vi "Iman.vi"() -> ()   [LabVIEW 2017]
uses:
  <vilib>/myRIO/Instrument Drivers/Onboard IO/DIO/typedefs/DIO Reference.ctl
  <vilib>/myRIO/Common/Instrument Driver Framework/Utilities/typedefs/myRIO Generic Hardware Reference.ctl
  <vilib>/myRIO/Common/Instrument Driver Framework/Utilities/typedefs/Hardware Version Enum.ctl
  <vilib>/myRIO/Common/Instrument Driver Framework/Utilities/typedefs/myRIO v1.0 Reference.ctl
  <vilib>/myRIO/Common/Instrument Driver Framework/Utilities/typedefs/Generic FPGA Reference.ctl
  <vilib>/myRIO/Common/Instrument Driver Framework/myRIO v1.0/DIO/typedefs/DIO Channels List.ctl
  <vilib>/myRIO/Common/Instrument Driver Framework/myRIO v1.0/DIO/typedefs/DIO Channels Enum.ctl
  <vilib>/userdefined/High Color/nirio_resource_hc.ctl
  <vilib>/myRIO/Common/Instrument Driver Framework/Utilities/vis/Is FPGA Ref Available.vi
  <vilib>/myRIO/Common/Instrument Driver Framework/myRIO v1.0/DIO/vis/myRIO v1.1 Open DIO.vi
  <vilib>/myRIO/Instrument Drivers/Onboard IO/DIO/vis/Write.vi
  <vilib>/myRIO/Common/Instrument Driver Framework/Utilities/vis/Validate Channels.vi
  <vilib>/myRIO/Common/Instrument Driver Framework/myRIO v1.0/DIO/vis/myRIO v1.0 Reserve DIO.vi
  <vilib>/myRIO/Common/Instrument Driver Framework/myRIO v1.0/Resource Manager/vis/myRIO v1.0 Reserve Channel List.vi
  <vilib>/myRIO/Common/Instrument Driver Framework/myRIO v1.0/DIO/vis/myRIO v1.0 Build MUX Configuration DIO.vi
  <vilib>/myRIO/Common/Instrument Driver Framework/myRIO v1.0/Resource Manager/vis/myRIO v1.0 Reserve Channel.vi
  <vilib>/myRIO/Common/Instrument Driver Framework/myRIO v1.0/Resource Manager/vis/myRIO v1.0 Unreserve Channel.vi
  <vilib>/myRIO/Common/Instrument Driver Framework/myRIO v1.0/Resource Manager/vis/myRIO v1.0 Create Configuration List.vi
  <vilib>/myRIO/Common/Instrument Driver Framework/myRIO v1.0/Resource Manager/vis/myRIO v1.0 Build Mutex Name.vi
  <vilib>/Utility/VariantDataType/GetNumericInfo.vi
  <vilib>/Utility/error.llb/Error Cluster From Error Code.vi
  <vilib>/myRIO/Common/Instrument Driver Framework/myRIO v1.0/myRIO v1.1 Open.vi
  <vilib>/myRIO/Common/Instrument Driver Framework/Utilities/vis/IO Manager.vi
  <vilib>/myRIO/Common/Instrument Driver Framework/Utilities/vis/Configuration Manager.vi
  <vilib>/myRIO/Common/Instrument Driver Framework/myRIO v1.0/Resource Manager/vis/myRIO v1.0 Configure IO.vi
  <vilib>/myRIO/Common/Instrument Driver Framework/myRIO v1.0/myRIO v1.0 Close.vi
  <vilib>/myRIO/Common/Instrument Driver Framework/myRIO v1.0/DIO/vis/myRIO v1.0 Write DIO.vi
  <vilib>/myRIO/Express VI/Onboard IO/DO/DO Express VI.xnode
  <vilib>/myRIO/Instrument Drivers/Onboard IO/DIO/vis/myRIO DIO Open.xnode
  <vilib>/myRIO/Express VI/Onboard Devices/LED/LED Express VI.xnode
  <vilib>/myRIO/Instrument Drivers/Onboard IO/DIO/DIO.lvlib
panel:
  out "array val":i32
  in  "Array 0-4":i32[](array[numeric])
  out "Segment":i32
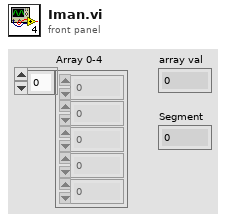
[diagram p1: front panel]
types:
  T1 = typedef "DIO.lvlib/DIO Reference.ctl" = cluster{"myRIO Reference":T2, "DIO Channels List":T6}
  T2 = typedef "myRIO Generic Hardware Reference.ctl" = cluster{"myRIO Model":T3, "myRIO Hardware Reference":T4}
  T3 = typedef "Hardware Version Enum.ctl" = enum16{"Unknown", "myRIO-1900", "myRIO-1950", "roboRIO", "NI ELVIS RIO CM"}
  T4 = typedef "myRIO v1.0 Reference.ctl" = cluster{"Generic FPGA Reference":T5, "Allow multiple opens":bool}
  T5 = typedef "Generic FPGA Reference.ctl" = refnum<k20>
  T6 = typedef "DIO Channels List.ctl" = T7[]
  T7 = typedef "DIO Channels Enum.ctl" = enum16{"Not Connected", "C/DIO0", "C/DIO1", "C/DIO2", "C/DIO3", "C/DIO4", "C/DIO5", "C/DIO6", "C/DIO7", "A/DIO0", "A/DIO1", "A/DIO2", "A/DIO3", "A/DIO4", "A/DIO5", "A/DIO6", "A/DIO7", "A/DIO8", "A/DIO9", "A/DIO10", "A/DIO11", "A/DIO12", "A/DIO13", "A/DIO14", "A/DIO15", "B/DIO0", "B/DIO1", "B/DIO2", "B/DIO3", "B/DIO4", "B/DIO5", "B/DIO6", "B/DIO7", "B/DIO8", "B/DIO9", "B/DIO10", "B/DIO11", "B/DIO12", "B/DIO13", "B/DIO14", "B/DIO15", "LED0", "LED1", "LED2", "LED3", "Button0", "DIO/DIO0", "DIO/DIO1", "DIO/DIO2", "DIO/DIO3", "DIO/DIO4", "DIO/DIO5", "DIO/DIO6", "DIO/DIO7", "DIO/DIO8", "DIO/DIO9", "SPI/CS0", "SPI/CS1", "SPI/CS2", "SPI/CS3", "LED RADIO (Green)", "LED RADIO (Red)", "LED COMM (Green)", "LED COMM (Red)", "LED MODE (Green)", "LED MODE (Red)"}
  T8 = typedef "nirio_resource_hc.ctl" = tag
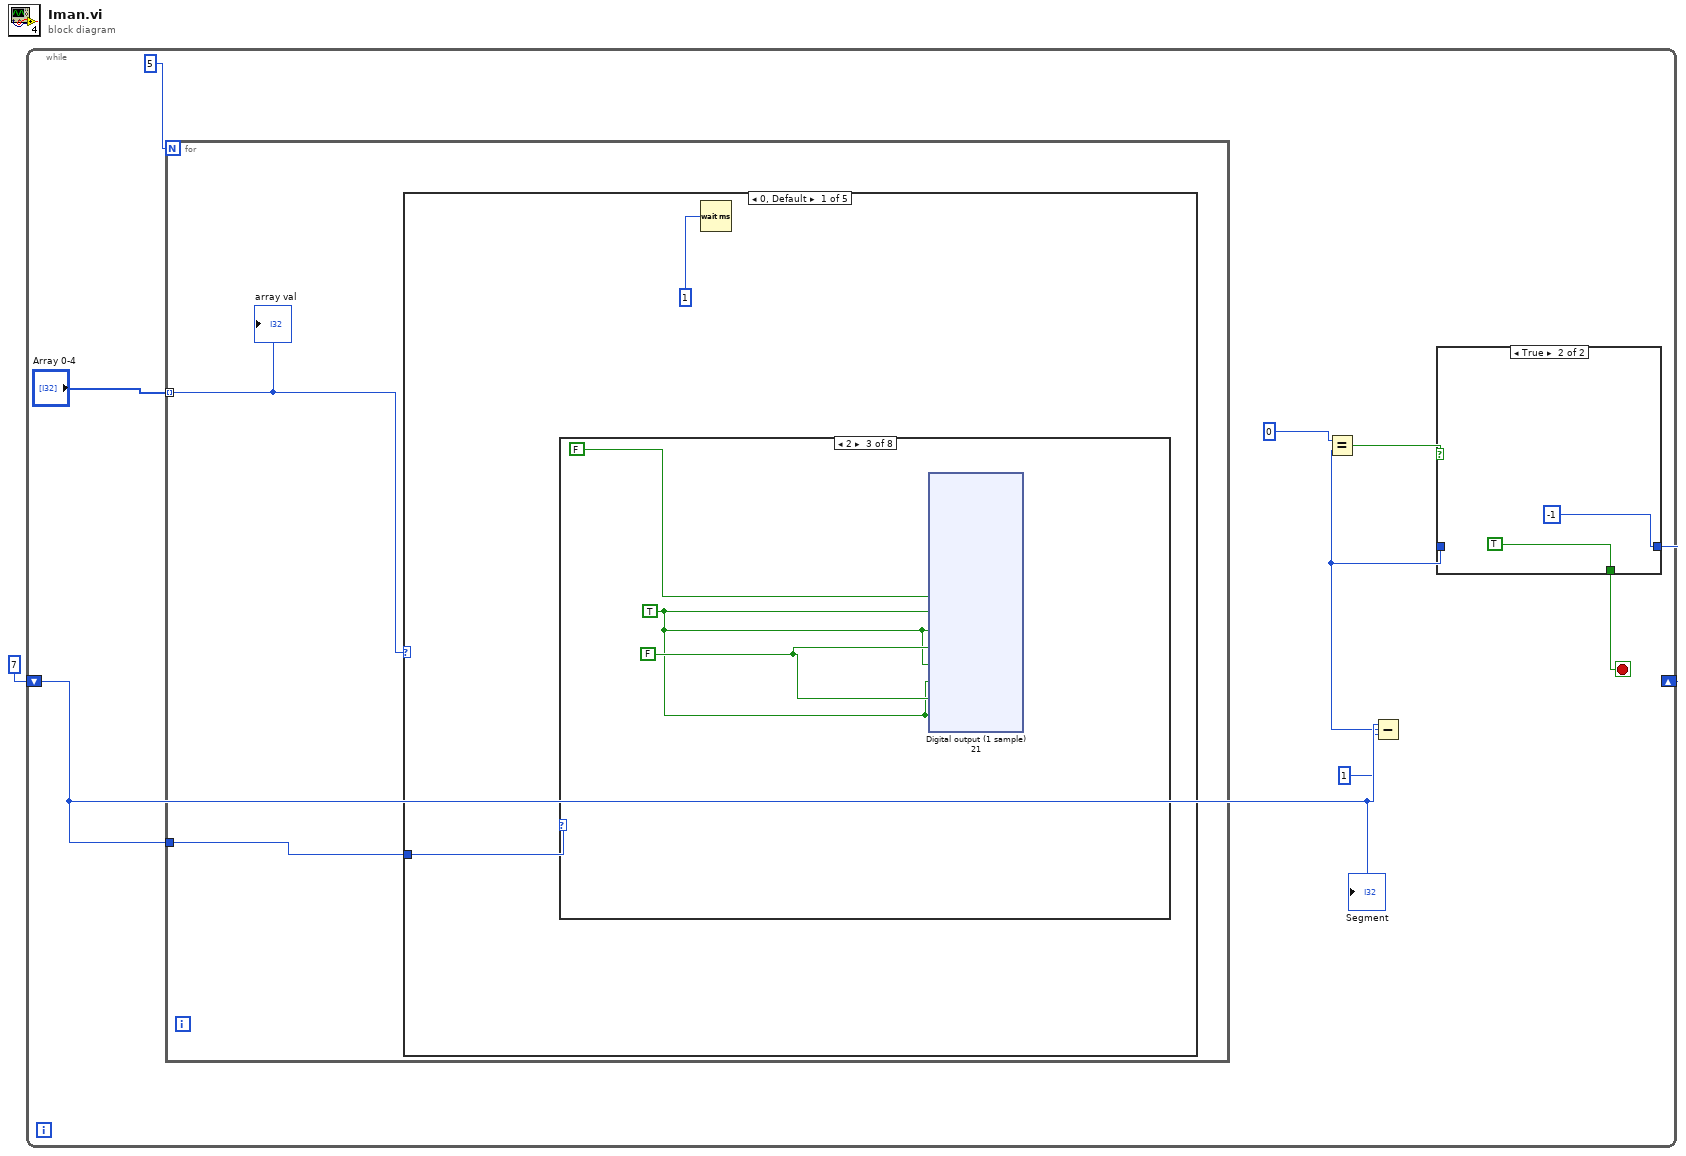
[diagram p0: block diagram]
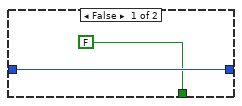
[diagram p2: hidden frame]
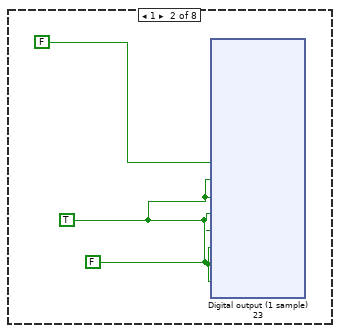
[diagram p4: hidden frame]
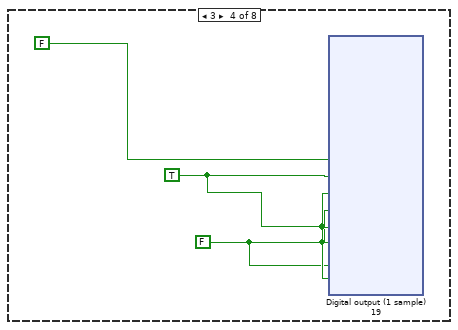
[diagram p5: hidden frame]
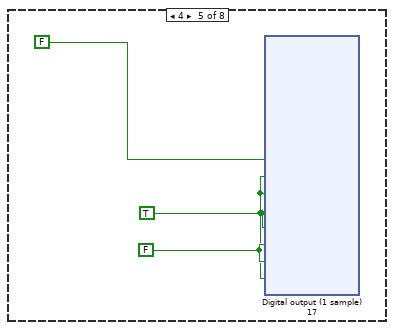
[diagram p6: hidden frame]
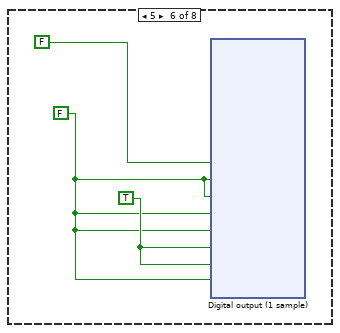
[diagram p7: hidden frame]
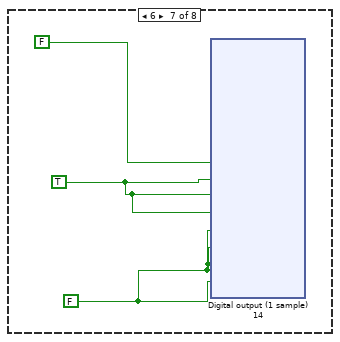
[diagram p8: hidden frame]
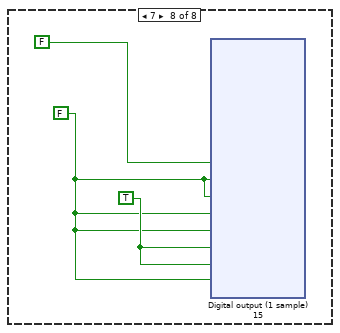
[diagram p9: hidden frame]
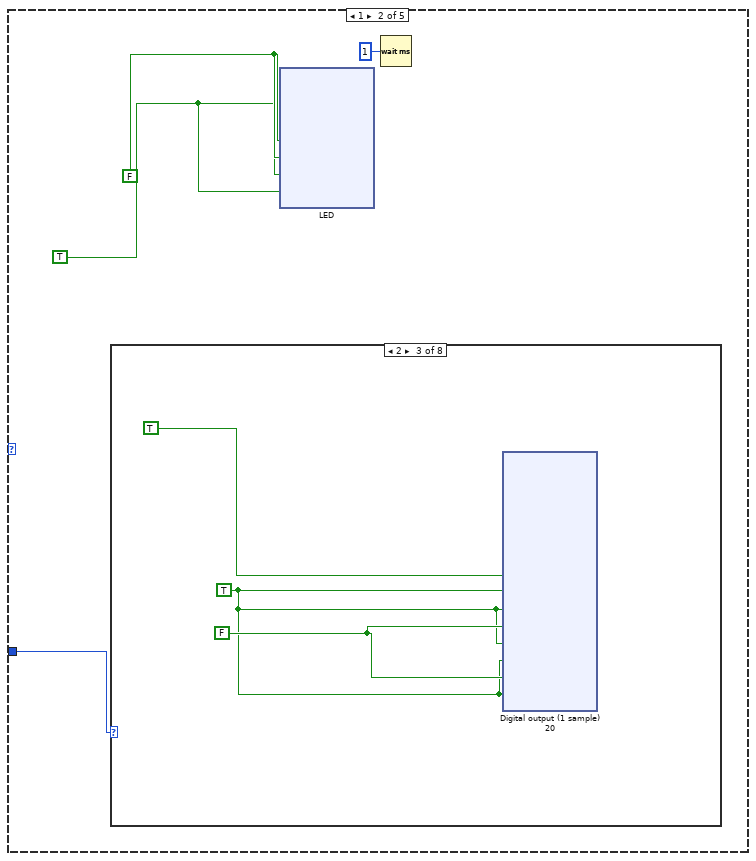
[diagram p10: hidden frame]
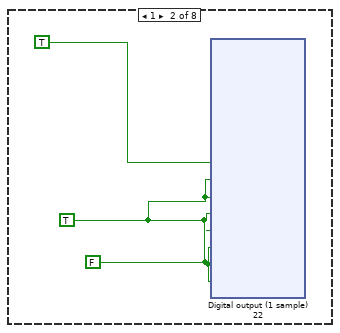
[diagram p12: hidden frame]
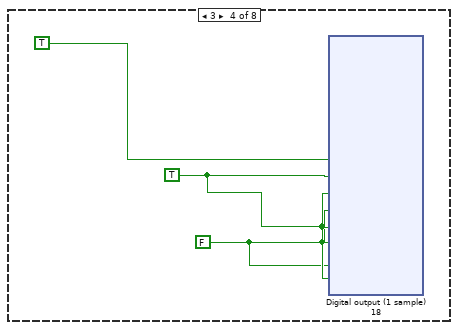
[diagram p13: hidden frame]
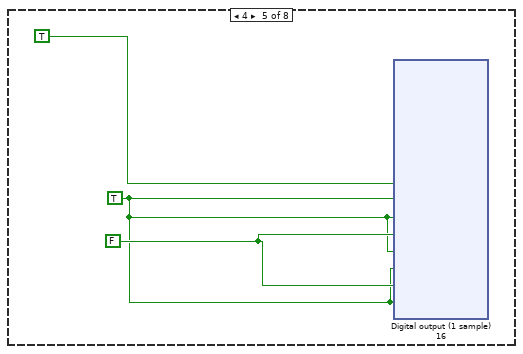
[diagram p14: hidden frame]
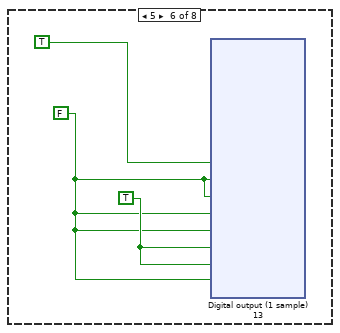
[diagram p15: hidden frame]
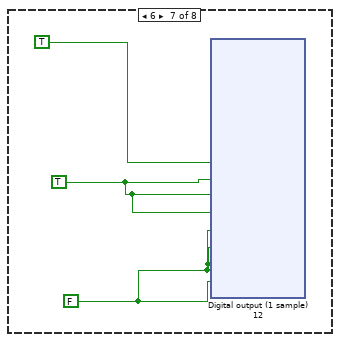
[diagram p16: hidden frame]
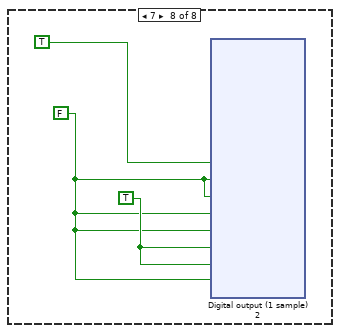
[diagram p17: hidden frame]
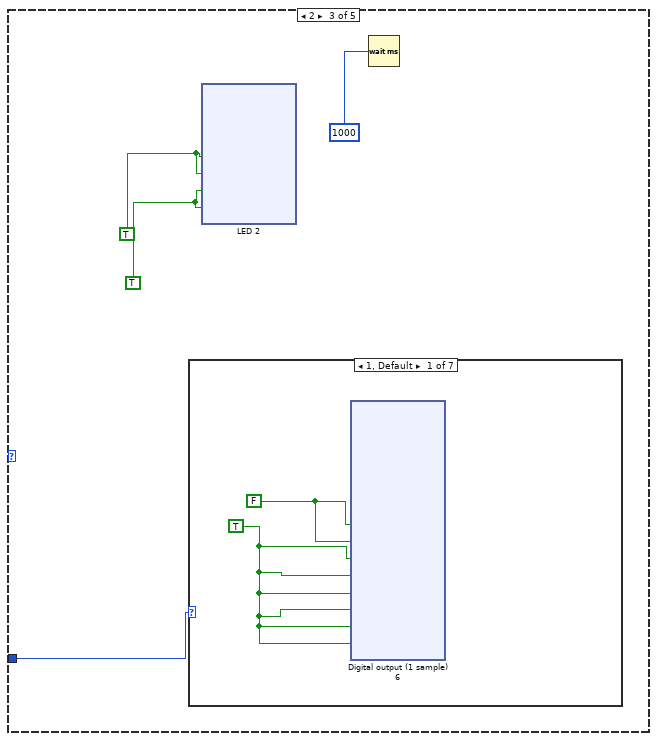
[diagram p18: hidden frame]
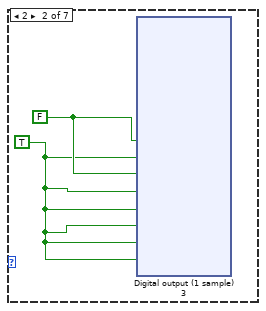
[diagram p19: hidden frame]
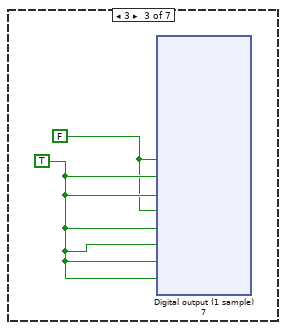
[diagram p20: hidden frame]
diagram:
  n1 = while {
    shift-right: [w3] -> _
    shift-left: 7 -> [w8]
    stop <- w2 stop-if-true
    n2 = for {
      N: 5 -> [_]
      tunnel: "Array 0-4" -> [w16] mode=indexing
      tunnel: w8 -> [w15]
      n3 = case shown="0, Default" w16 {
        tunnel: w15 -> [w17 w334 w692 _ _]
        frame 0, Default {
          n4 = case shown="2" w17 {
            frame 0, Default {
            }
            frame 1 {
              w19 = FALSE
              w20 = TRUE
              n5 = xnode "Digital output (1 sample) 23"("A/DIO7 (Pin 25)"=FALSE, "A/DIO0 (Pin 11)"=w20, "A/DIO1 (Pin 13)"=w20, "A/DIO2 (Pin 15)"=w20, "A/DIO3 (Pin 17)"=w19, "A/DIO4 (Pin 19)"=w19, "A/DIO5 (Pin 21)"=w20, "A/DIO6 (Pin 23)"=w20) -> ()  [unwired: 1 in, 1 out]
            }
            frame 2 {
              w64 = TRUE
              w65 = FALSE
              n6 = xnode "Digital output (1 sample) 21"("A/DIO7 (Pin 25)"=FALSE, "A/DIO0 (Pin 11)"=w64, "A/DIO1 (Pin 13)"=w64, "A/DIO2 (Pin 15)"=w65, "A/DIO3 (Pin 17)"=w64, "A/DIO4 (Pin 19)"=w64, "A/DIO5 (Pin 21)"=w65, "A/DIO6 (Pin 23)"=w64) -> ()  [unwired: 1 in, 1 out]
            }
            frame 3 {
              w109 = FALSE
              w110 = TRUE
              n7 = xnode "Digital output (1 sample) 19"("A/DIO7 (Pin 25)"=FALSE, "A/DIO0 (Pin 11)"=w110, "A/DIO1 (Pin 13)"=w110, "A/DIO2 (Pin 15)"=w109, "A/DIO3 (Pin 17)"=w110, "A/DIO4 (Pin 19)"=w110, "A/DIO5 (Pin 21)"=w109, "A/DIO6 (Pin 23)"=w110) -> ()  [unwired: 1 in, 1 out]
            }
            frame 4 {
              w154 = TRUE
              w155 = FALSE
              n8 = xnode "Digital output (1 sample) 17"("A/DIO7 (Pin 25)"=FALSE, "A/DIO0 (Pin 11)"=w154, "A/DIO1 (Pin 13)"=w154, "A/DIO2 (Pin 15)"=w154, "A/DIO3 (Pin 17)"=w154, "A/DIO4 (Pin 19)"=w155, "A/DIO5 (Pin 21)"=w155, "A/DIO6 (Pin 23)"=w154) -> ()  [unwired: 1 in, 1 out]
            }
            frame 5 {
              w200 = TRUE
              w199 = FALSE
              n9 = xnode "Digital output (1 sample)"("A/DIO7 (Pin 25)"=FALSE, "A/DIO0 (Pin 11)"=w199, "A/DIO1 (Pin 13)"=w199, "A/DIO2 (Pin 15)"=w199, "A/DIO3 (Pin 17)"=w199, "A/DIO4 (Pin 19)"=w200, "A/DIO5 (Pin 21)"=w200, "A/DIO6 (Pin 23)"=w199) -> ()  [unwired: 1 in, 1 out]
            }
            frame 6 {
              w244 = FALSE
              w245 = TRUE
              n10 = xnode "Digital output (1 sample) 14"("A/DIO7 (Pin 25)"=FALSE, "A/DIO0 (Pin 11)"=w245, "A/DIO1 (Pin 13)"=w245, "A/DIO2 (Pin 15)"=w245, "A/DIO3 (Pin 17)"=w244, "A/DIO4 (Pin 19)"=w244, "A/DIO5 (Pin 21)"=w244, "A/DIO6 (Pin 23)"=w244) -> ()  [unwired: 1 in, 1 out]
            }
            frame 7 {
              w290 = TRUE
              w289 = FALSE
              n11 = xnode "Digital output (1 sample) 15"("A/DIO7 (Pin 25)"=FALSE, "A/DIO0 (Pin 11)"=w289, "A/DIO1 (Pin 13)"=w289, "A/DIO2 (Pin 15)"=w289, "A/DIO3 (Pin 17)"=w289, "A/DIO4 (Pin 19)"=w290, "A/DIO5 (Pin 21)"=w290, "A/DIO6 (Pin 23)"=w289) -> ()  [unwired: 1 in, 1 out]
            }
          }
          n12 = Wait (ms)(milliseconds to wait=u32 1) -> ()  [unwired: 1 out]
        }
        frame 1 {
          w336 = TRUE
          w337 = FALSE
          n13 = case shown="2" w334 {
            frame 0, Default {
            }
            frame 1 {
              w338 = FALSE
              w339 = TRUE
              n14 = xnode "Digital output (1 sample) 22"("A/DIO7 (Pin 25)"=TRUE, "A/DIO0 (Pin 11)"=w339, "A/DIO1 (Pin 13)"=w339, "A/DIO2 (Pin 15)"=w339, "A/DIO3 (Pin 17)"=w338, "A/DIO4 (Pin 19)"=w338, "A/DIO5 (Pin 21)"=w339, "A/DIO6 (Pin 23)"=w339) -> ()  [unwired: 1 in, 1 out]
            }
            frame 2 {
              w383 = TRUE
              w384 = FALSE
              n15 = xnode "Digital output (1 sample) 20"("A/DIO7 (Pin 25)"=TRUE, "A/DIO0 (Pin 11)"=w383, "A/DIO1 (Pin 13)"=w383, "A/DIO2 (Pin 15)"=w384, "A/DIO3 (Pin 17)"=w383, "A/DIO4 (Pin 19)"=w383, "A/DIO5 (Pin 21)"=w384, "A/DIO6 (Pin 23)"=w383) -> ()  [unwired: 1 in, 1 out]
            }
            frame 3 {
              w428 = FALSE
              w429 = TRUE
              n16 = xnode "Digital output (1 sample) 18"("A/DIO7 (Pin 25)"=TRUE, "A/DIO0 (Pin 11)"=w429, "A/DIO1 (Pin 13)"=w429, "A/DIO2 (Pin 15)"=w428, "A/DIO3 (Pin 17)"=w429, "A/DIO4 (Pin 19)"=w429, "A/DIO5 (Pin 21)"=w428, "A/DIO6 (Pin 23)"=w429) -> ()  [unwired: 1 in, 1 out]
            }
            frame 4 {
              w473 = TRUE
              w474 = FALSE
              n17 = xnode "Digital output (1 sample) 16"("A/DIO7 (Pin 25)"=TRUE, "A/DIO0 (Pin 11)"=w473, "A/DIO1 (Pin 13)"=w473, "A/DIO2 (Pin 15)"=w474, "A/DIO3 (Pin 17)"=w473, "A/DIO4 (Pin 19)"=w473, "A/DIO5 (Pin 21)"=w474, "A/DIO6 (Pin 23)"=w473) -> ()  [unwired: 1 in, 1 out]
            }
            frame 5 {
              w519 = TRUE
              w518 = FALSE
              n18 = xnode "Digital output (1 sample) 13"("A/DIO7 (Pin 25)"=TRUE, "A/DIO0 (Pin 11)"=w518, "A/DIO1 (Pin 13)"=w518, "A/DIO2 (Pin 15)"=w518, "A/DIO3 (Pin 17)"=w518, "A/DIO4 (Pin 19)"=w519, "A/DIO5 (Pin 21)"=w519, "A/DIO6 (Pin 23)"=w518) -> ()  [unwired: 1 in, 1 out]
            }
            frame 6 {
              w563 = FALSE
              w564 = TRUE
              n19 = xnode "Digital output (1 sample) 12"("A/DIO7 (Pin 25)"=TRUE, "A/DIO0 (Pin 11)"=w564, "A/DIO1 (Pin 13)"=w564, "A/DIO2 (Pin 15)"=w564, "A/DIO3 (Pin 17)"=w563, "A/DIO4 (Pin 19)"=w563, "A/DIO5 (Pin 21)"=w563, "A/DIO6 (Pin 23)"=w563) -> ()  [unwired: 1 in, 1 out]
            }
            frame 7 {
              w609 = TRUE
              w608 = FALSE
              n20 = xnode "Digital output (1 sample) 2"("A/DIO7 (Pin 25)"=TRUE, "A/DIO0 (Pin 11)"=w608, "A/DIO1 (Pin 13)"=w608, "A/DIO2 (Pin 15)"=w608, "A/DIO3 (Pin 17)"=w608, "A/DIO4 (Pin 19)"=w609, "A/DIO5 (Pin 21)"=w609, "A/DIO6 (Pin 23)"=w608) -> ()  [unwired: 1 in, 1 out]
            }
          }
          n21 = xnode "LED"("LED0"=w337, "LED1"=w337, "LED2"=w336, "LED3"=w336) -> ()  [unwired: 1 in, 1 out]
          n22 = Wait (ms)(milliseconds to wait=u32 1) -> ()  [unwired: 1 out]
        }
        frame 2 {
          w693 = TRUE
          w694 = TRUE
          n23 = case shown="1, Default" w692 {
            frame 1, Default {
              w695 = FALSE
              w696 = TRUE
              n24 = xnode "Digital output (1 sample) 6"("A/DIO7 (Pin 25)"=w695, "A/DIO0 (Pin 11)"=w695, "A/DIO1 (Pin 13)"=w696, "A/DIO2 (Pin 15)"=w696, "A/DIO3 (Pin 17)"=w696, "A/DIO4 (Pin 19)"=w696, "A/DIO5 (Pin 21)"=w696, "A/DIO6 (Pin 23)"=w696) -> ()  [unwired: 1 in, 1 out]
            }
            frame 2 {
              w740 = FALSE
              w739 = TRUE
              n25 = xnode "Digital output (1 sample) 3"("A/DIO7 (Pin 25)"=w740, "A/DIO0 (Pin 11)"=w739, "A/DIO1 (Pin 13)"=w740, "A/DIO2 (Pin 15)"=w739, "A/DIO3 (Pin 17)"=w739, "A/DIO4 (Pin 19)"=w739, "A/DIO5 (Pin 21)"=w739, "A/DIO6 (Pin 23)"=w739) -> ()  [unwired: 1 in, 1 out]
            }
            frame 3 {
              w783 = FALSE
              w784 = TRUE
              n26 = xnode "Digital output (1 sample) 7"("A/DIO7 (Pin 25)"=w783, "A/DIO0 (Pin 11)"=w784, "A/DIO1 (Pin 13)"=w784, "A/DIO2 (Pin 15)"=w783, "A/DIO3 (Pin 17)"=w784, "A/DIO4 (Pin 19)"=w784, "A/DIO5 (Pin 21)"=w784, "A/DIO6 (Pin 23)"=w784) -> ()  [unwired: 1 in, 1 out]
            }
            frame 4 {
              w827 = FALSE
              w828 = TRUE
              n27 = xnode "Digital output (1 sample) 8"("A/DIO7 (Pin 25)"=w827, "A/DIO0 (Pin 11)"=w828, "A/DIO1 (Pin 13)"=w828, "A/DIO2 (Pin 15)"=w828, "A/DIO3 (Pin 17)"=w827, "A/DIO4 (Pin 19)"=w828, "A/DIO5 (Pin 21)"=w828, "A/DIO6 (Pin 23)"=w828) -> ()  [unwired: 1 in, 1 out]
            }
            frame 5 {
              w871 = FALSE
              w872 = TRUE
              n28 = xnode "Digital output (1 sample) 9"("A/DIO7 (Pin 25)"=w871, "A/DIO0 (Pin 11)"=w872, "A/DIO1 (Pin 13)"=w872, "A/DIO2 (Pin 15)"=w872, "A/DIO3 (Pin 17)"=w872, "A/DIO4 (Pin 19)"=w871, "A/DIO5 (Pin 21)"=w872, "A/DIO6 (Pin 23)"=w872) -> ()  [unwired: 1 in, 1 out]
            }
            frame 6 {
              w915 = FALSE
              w916 = TRUE
              n29 = xnode "Digital output (1 sample) 10"("A/DIO7 (Pin 25)"=w915, "A/DIO0 (Pin 11)"=w916, "A/DIO1 (Pin 13)"=w916, "A/DIO2 (Pin 15)"=w916, "A/DIO3 (Pin 17)"=w916, "A/DIO4 (Pin 19)"=w916, "A/DIO5 (Pin 21)"=w915, "A/DIO6 (Pin 23)"=w916) -> ()  [unwired: 1 in, 1 out]
            }
            frame 7 {
              w959 = FALSE
              w960 = TRUE
              n30 = xnode "Digital output (1 sample) 11"("A/DIO7 (Pin 25)"=w959, "A/DIO0 (Pin 11)"=w960, "A/DIO1 (Pin 13)"=w960, "A/DIO2 (Pin 15)"=w960, "A/DIO3 (Pin 17)"=w960, "A/DIO4 (Pin 19)"=w960, "A/DIO5 (Pin 21)"=w960, "A/DIO6 (Pin 23)"=w959) -> ()  [unwired: 1 in, 1 out]
            }
          }
          n31 = xnode "LED 2"("LED0"=w694, "LED1"=w694, "LED2"=w693, "LED3"=w693) -> ()  [unwired: 1 in, 1 out]
          n32 = Wait (ms)(milliseconds to wait=u32 1000) -> ()  [unwired: 1 out]
        }
        frame 3 {
          w1044 = FALSE ("A/DIO6 (Pin 23)")
          w1043 = FALSE
          n33 = xnode "Digital output (1 sample) 4"("A/DIO7 (Pin 25)"=TRUE, "A/DIO0 (Pin 11)"=w1043, "A/DIO1 (Pin 13)"=w1043, "A/DIO2 (Pin 15)"=w1043, "A/DIO3 (Pin 17)"=w1043, "A/DIO4 (Pin 19)"=w1044, "A/DIO5 (Pin 21)"=w1044, "A/DIO6 (Pin 23)"=w1043) -> ()  [unwired: 1 in, 1 out]
          n34 = Wait (ms)(milliseconds to wait=u32 1) -> ()  [unwired: 1 out]
        }
        frame 4 {
          w1088 = TRUE
          n35 = xnode "Digital output (1 sample) 5"("A/DIO7 (Pin 25)"=FALSE, "A/DIO0 (Pin 11)"=w1088, "A/DIO1 (Pin 13)"=w1088, "A/DIO2 (Pin 15)"=w1088, "A/DIO3 (Pin 17)"=w1088, "A/DIO4 (Pin 19)"=w1088, "A/DIO5 (Pin 21)"=w1088, "A/DIO6 (Pin 23)"=w1088) -> ()  [unwired: 1 in, 1 out]
          n36 = Wait (ms)(milliseconds to wait=u32 1) -> ()  [unwired: 1 out]
        }
      }
      "array val" <- w16
    }
    n37 = Subtract(x=w8, y=1) -> (x-y=w4:i32)
    n38 = Equal?(x=0, y=w4) -> (x = y?=w5:bool)
    n39 = case shown="True" w5 {
      tunnel: w4 -> [w12 _]
      tunnel: [w12 -1] -> w3
      tunnel: [FALSE TRUE] -> w2
      frame False {
      }
      frame True {
      }
    }
    "Segment" <- w8
  }
